vi "RSZVB Get Session Info.vi"(8 "error in (no error)":errorcluster {"code" format="%.0x"}, 11 "VISA session":refnum<visa-resource-name>) -> (0 "error out":errorcluster {"code" format="%.0x"}, 1 "Session Info":T1, 3 "dup VISA session":refnum<visa-resource-name>)   [LabVIEW 2015]
doc: "This VI reads data from the instrument's output buffer and returns it to the specified variable in memory.\n\nNotes:\n\n(1) Because the instrument may return both numeric and text data in response to queries this VI returns the data in string format.\n\n(2) If valid data is not available at the instrument's output buffer when this VI is called the instrument will hang up and the function will not return until it times out. If the time-out is disabled this function will hang indefinitely and it may be necessary to reboot the computer to break out."
uses:
  RSZVB Global Data.vi
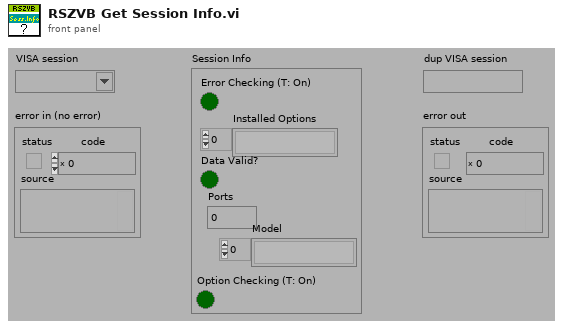
[diagram p1: front panel]
types:
  T1 = cluster{"Error Checking (T: On)":bool, "Installed Options":string[], "Data Valid?":bool, "Ports":i32, "Model":string[], "Option Checking (T: On)":bool}
  T2 = cluster{"Error Checking (T: On)":bool, "Installed Options":string[], "Data Valid?":bool, "Ports":i32, "Model":string[], "Option Checking (T: On)":bool}[]
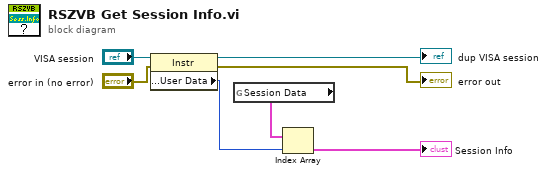
[diagram p0: block diagram]
diagram:
  n1 = property class="Instr"(reference="VISA session", error in="error in (no error)") -> (reference out=→"dup VISA session":refnum<visa-resource-name>, error out=→"error out":errorcluster, "General Settings:User Data"=w5:u32)
  n2 = global read "RSZVB Global Data.vi" "Session Data"() -> (w1:T2)
  n3 = Index Array(array=w1, index=w5) -> (element=→"Session Info":T1)
